vi "Setup.vi"(0 "Test Label":string, 11 "error in":errorcluster) -> (4 "Application Ref":refnum<vi>, 6 "VI Reference Out":refnum<vi>, 15 "error out":errorcluster)   [LabVIEW 2016, in "Drona.lvlib"]
doc: "Initiates the launcher VI as specified in Drona configuration file and return its application & VI reference."
uses:
  Drona.lvlib
  _Typedefs/SetupSourceConfig.ctl
  _Typedefs/SetupEXEConfig.ctl
  <vilib>/Utility/error.llb/Error Cluster From Error Code.vi
  Get/GetVI/GetVIByPath.vi
  Stimulus/VI/OpenVIFrontPanel.vi
  Stimulus/VI/RunVI.vi
  Get/GetVI/GetVIByName.vi
  <vilib>/ErrorRing/Error Ring.xnode
  Get/GetVI/GetVI.lvlib
  <vilib>/Utility/config.llb/NI_LVConfig.lvlib
  <vilib>/SLL Toolkit/SLL File IO/SLL File IO.lvlib
  Stimulus/VI/VI.lvlib
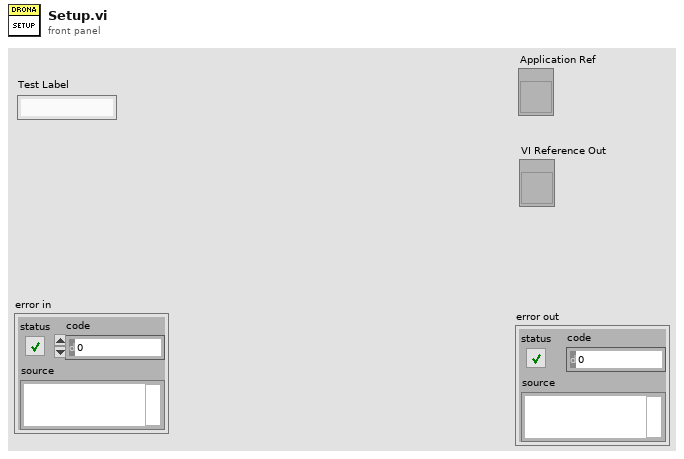
[diagram p1: front panel]
types:
  T1 = typedef "Drona.lvlib/SetupSourceConfig.ctl" = cluster{"LauncherPath":path, "Open?":bool, "Run?":bool}
  T2 = typedef "NI_LVConfig.lvlib/Config Data RefNum.ctl" = refnum<k1>
  T3 = enum32{"Bad", "Idle", "Run top level", "Running"}
  T4 = typedef "Drona.lvlib/SetupEXEConfig.ctl" = cluster{"LauncherName":string}
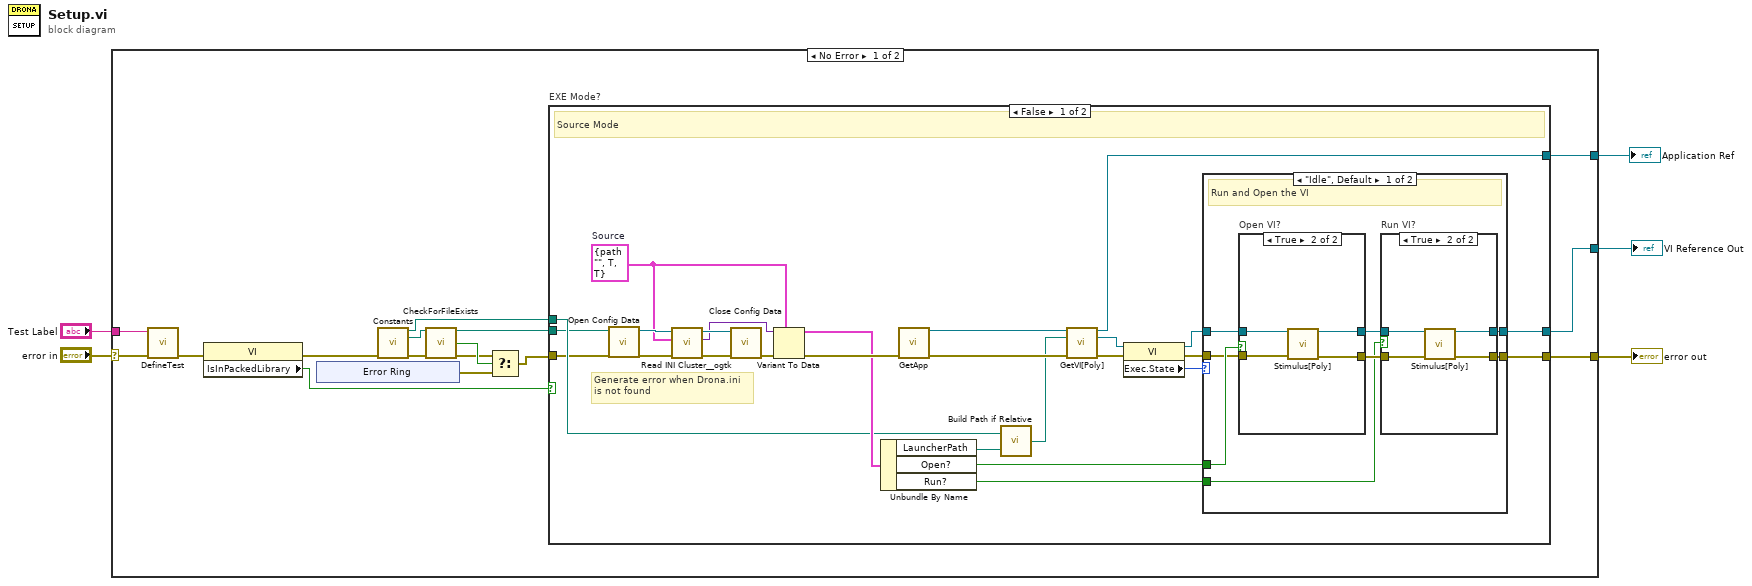
[diagram p0: block diagram]
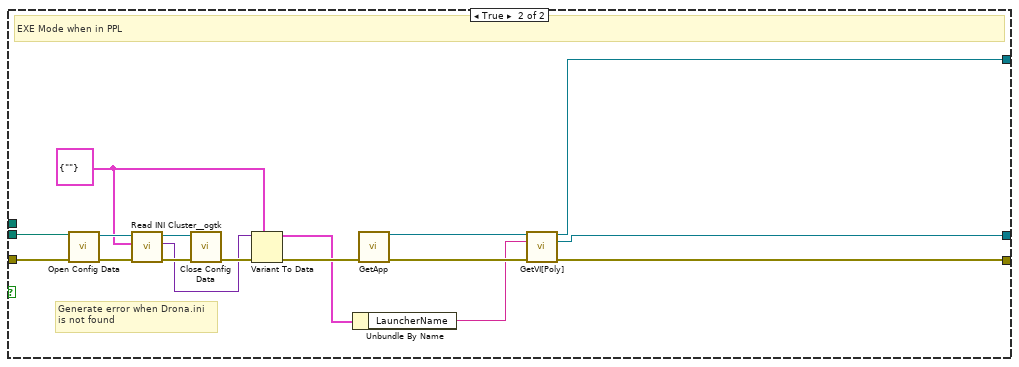
[diagram p5: hidden frame]
diagram:
  n1 = case shown="No Error" "error in" {
    selector: "error in" -> [w8 w92]
    tunnel: [w21 _] -> w4
    tunnel: [w20 _] -> w3
    tunnel: [w19 w92] -> w2
    tunnel: "Test Label" -> [w6 _]
    frame No Error {
      n2 = call "DefineTest.vi"("Test Label"=w6, "error in (no error)"=w8) -> ("error out"=w7:errorcluster)  [unwired: 13 in]
      n3 = property class="VI"(error in=w7) -> (error out=w17:errorcluster, "IsInPackedLibrary"=w18:bool)  [unwired: 1 in, 1 out]
      n4 = xnode "Error Ring"() -> ("error out"=w13:errorcluster)
      n5 = call "Constants.vi"("error in"=w17) -> ("Source path"=w9:path, "Drona ini file path"=w10:path, "error out"=w16:errorcluster)  [unwired: 12 in]
      n6 = call "CheckForFileExists.vi"("Path"=w10, "error in"=w16) -> ("Dup Path"=w15:path, "File Exists?"=w14:bool, "error out"=w12:errorcluster)  [unwired: 11 in]
      n7 = Select(t=w12, s=w14, f=w13) -> (s? t:f=w11:errorcluster)
      n8 = case "EXE Mode?" shown="False" w18 {
        tunnel: [w47 w86] -> w21
        tunnel: [w46 w85] -> w20
        tunnel: [w45 w89] -> w19
        tunnel: w11 -> [w27 w76]
        tunnel: w15 -> [w28 w75]
        tunnel: w9 -> [w29 _]
        frame False {
          w30 = T1 {"LauncherPath"=path "", "Open?"=TRUE, "Run?"=TRUE}  # Source
          # "Generate error when Drona.ini\nis not found"
          # "Source Mode"
          n9 = call <vilib>:"Open Config Data.vi"("error in (no error)"=w27, "configuration file path"=w28) -> ("error out"=w35:errorcluster, "refnum"=w34:T2)  [unwired: 7 in, 1 out]
          n10 = call <userlib>:"Read INI Cluster__ogtk.vi"("error in (no error)"=w35, "INI Fomatted Cluster Type"=w30, "refnum"=w34) -> ("error out"=w36:errorcluster, "INI Fomatted Cluster"=w31:variant, "dup refnum"=w32:T2)  [unwired: 4 in, 2 out]
          n11 = call <vilib>:"Close Config Data.vi"("error in (no error)"=w36, "refnum"=w32) -> ("error out"=w33:errorcluster)  [unwired: 8 in, 1 out]
          n12 = Variant To Data(error in=w33, type=w30, Variant=w31) -> (data=w48:T1, error out=w49:errorcluster)
          n13 = Unbundle By Name(w48) -> ("LauncherPath"=w38:path, "Open?"=w44:bool, "Run?"=w43:bool)
          n14 = call "GetApp.vi"("error in (no error)"=w49) -> ("Application Ref"=w51:refnum<vi>, "error out"=w52:errorcluster)  [unwired: 13 in]
          n15 = call <vilib>:"Build Path if Relative.vi"("Relative or Absolute Path"=w38, "Base Path"=w29) -> ("Path Out"=w37:path)
          n16 = call-poly "GetVI[Poly].vi"("Application Ref in"=w51, "VI Path"=w37, "error in (no error)"=w52) -> ("Application Ref out"=w47:refnum<vi>, "VI Reference"=w41:refnum<vi>, "error out"=w50:errorcluster)  [unwired: 10 in]
          n17 = property class="VI"(reference=w41, error in=w50) -> (reference out=w40:refnum<vi>, error out=w42:errorcluster, "Exec.State"=w39:T3)
          n18 = case shown="\"Idle\", Default" w39 {
            tunnel: [w58 w73] -> w46
            tunnel: [w57 w74] -> w45
            tunnel: w44 -> [w56 _]
            tunnel: w43 -> [w55 _]
            tunnel: w42 -> [w54 w74]
            tunnel: w40 -> [w53 w73]
            frame "Idle", Default {
              # "Run and Open the VI"
              n19 = case "Open VI?" shown="True" w56 {
                tunnel: [w67 w69] -> w60
                tunnel: [w68 w71] -> w59
                tunnel: w54 -> [w67 w70]
                tunnel: w53 -> [w68 w72]
                frame False {
                }
                frame True {
                  n20 = call-poly "Stimulus[Poly].vi"("VI Reference In"=w72, "error in"=w70) -> ("VI Reference Out"=w71:refnum<vi>, "error out"=w69:errorcluster)  [unwired: 12 in]
                }
              }
              n21 = case "Run VI?" shown="True" w55 {
                tunnel: w60 -> [w61 w65]
                tunnel: w59 -> [w62 w66]
                tunnel: [w62 w64] -> w58
                tunnel: [w61 w63] -> w57
                frame False {
                }
                frame True {
                  n22 = call-poly "Stimulus[Poly].vi"("VI Reference In"=w66, "error in"=w65) -> ("VI Reference Out"=w64:refnum<vi>, "error out"=w63:errorcluster)  [unwired: 12 in]
                }
              }
            }
            frame "Run top level" {
              # "Already Running"
            }
          }
        }
        frame True {
          w77 = T4 {"LauncherName"=""} ("EXE")
          # "Generate error when Drona.ini\nis not found"
          # "EXE Mode when in PPL"
          n23 = call <vilib>:"Open Config Data.vi"("error in (no error)"=w76, "configuration file path"=w75) -> ("error out"=w82:errorcluster, "refnum"=w81:T2)  [unwired: 7 in, 1 out]
          n24 = call <userlib>:"Read INI Cluster__ogtk.vi"("error in (no error)"=w82, "INI Fomatted Cluster Type"=w77, "refnum"=w81) -> ("error out"=w83:errorcluster, "INI Fomatted Cluster"=w78:variant, "dup refnum"=w79:T2)  [unwired: 4 in, 2 out]
          n25 = call <vilib>:"Close Config Data.vi"("error in (no error)"=w83, "refnum"=w79) -> ("error out"=w80:errorcluster)  [unwired: 8 in, 1 out]
          n26 = Variant To Data(error in=w80, type=w77, Variant=w78) -> (data=w87:T4, error out=w88:errorcluster)
          n27 = Unbundle By Name(w87) -> ("LauncherName"=w84:string)
          n28 = call "GetApp.vi"("error in (no error)"=w88) -> ("Application Ref"=w90:refnum<vi>, "error out"=w91:errorcluster)  [unwired: 13 in]
          n29 = call-poly "GetVI[Poly].vi"("Application Ref in"=w90, "VI Name"=w84, "error in (no error)"=w91) -> ("Application Ref out"=w86:refnum<vi>, "VI Reference"=w85:refnum<vi>, "error out"=w89:errorcluster)  [unwired: 10 in]
        }
      }
    }
    frame Error {
    }
  }
  "error out" <- w2
  "VI Reference Out" <- w3
  "Application Ref" <- w4
